vi "Read Serial Number.vi"(11 "Instrument in":refnum<class "Instrument.lvclass">) -> (2 "Serial Number":string, 3 "Instrument out":refnum<class "Instrument.lvclass">)   [LabVIEW 2020, in "Instrument.lvclass"]
uses:
  Instrument.lvclass
  Instrument.lvclass/Instrument.ctl
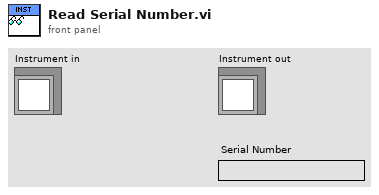
[diagram p1: front panel]
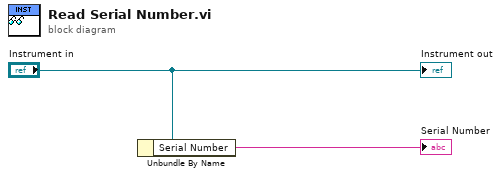
[diagram p0: block diagram]
diagram:
  n1 = Unbundle By Name("Instrument in") -> ("Serial Number"=→"Serial Number":string)
  "Instrument out" <- "Instrument in"
